vi "Verify Monotonicity.vi"(1 "Data In":string[][](array[string])) -> (0 "Monotonicity":bool)   [LabVIEW 2010]
panel:
  in  "disabled index (col)":i32
  in  "Test Data Array 1":dbl[][](array[numeric])=[[1.0, 20000.0], [2.0, 3000.0], [3.0, 400.0], [4.0, 50.0], [5.0, 6.0], [6.0, 1.0]]
  in  "Test Data Array 2":dbl[][](array[numeric])=[[1.0, 2.0], [2.0, 30.0], [3.0, 400.0], [4.0, 5000.0], [5.0, 60000.0], [6.0, 100000.0]]
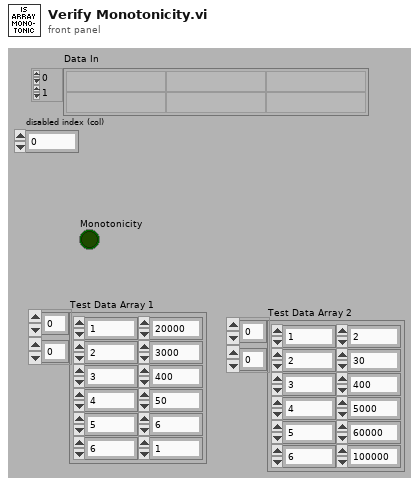
[diagram p1: front panel]
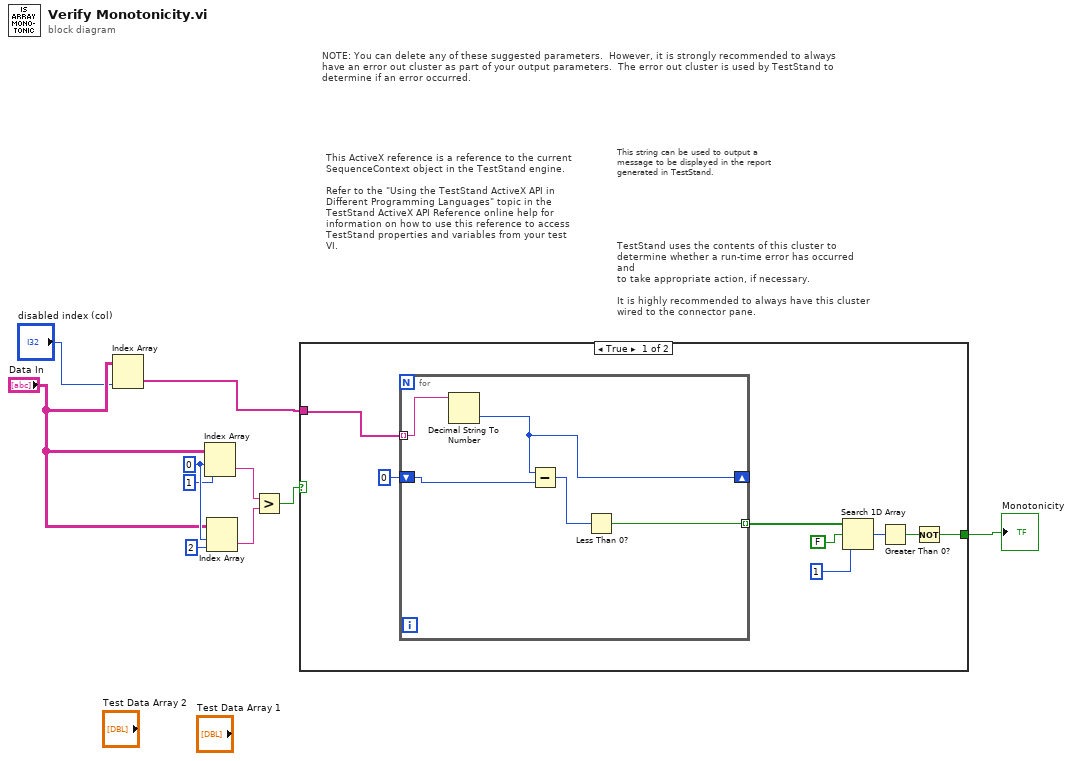
[diagram p0: block diagram]
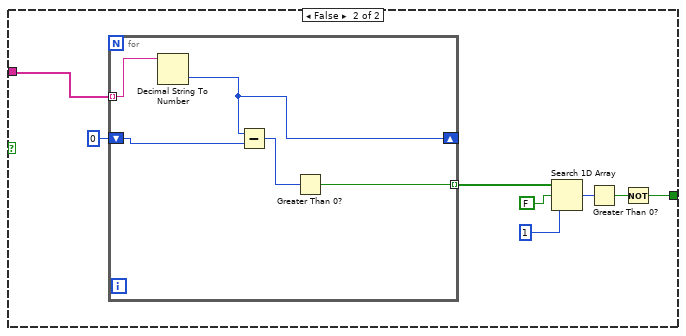
[diagram p2: hidden frame]
diagram:
  w6 = 0 ("index (row)")
  # "TestStand uses the contents of this cluster to\ndetermine whether a run-time error has occurred and\nto take appropriate action, if necessary.\n\nIt is highly recommended to always have this cluster\nwired to the connector pane."
  # "This string can be used to output a\nmessage to be displayed in the report\ngenerated in TestStand."
  # "NOTE: You can delete any of these suggested parameters.  However, it is strongly recommended to always have an error out cluster as part of your output parameters.  The error out cluster is used by TestStand to determine if an error occurred."
  # "This ActiveX reference is a reference to the current\nSequenceContext object in the TestStand engine.\n\nRefer to the \"Using the TestStand ActiveX API in\nDifferent Programming Languages\" topic in the \nTestStand ActiveX API Reference online help for\ninformation on how to use this reference to access\nTestStand properties and variables from your test VI."
  n1 = Index Array(array="Data In", index (col)="disabled index (col)") -> (element=w1:string[])  [unwired: 1 in]
  n2 = Index Array(array="Data In", index (row)=w6, index (col)=1 ("disabled index (col)")) -> (element=w10:string)
  n3 = Index Array(array="Data In", index (row)=w6, index (col)=2 ("disabled index (col)")) -> (element=w9:string)
  n4 = Greater?(x=w10, y=w9) -> (0:w8:bool)
  n5 = case shown="True" w8 {
    tunnel: w1 -> [w18 w31]
    tunnel: [w14 w27] -> w7
    frame True {
      n6 = for {
        tunnel: w18 -> [w21] mode=indexing
        tunnel: [w22] -> w13 mode=indexing
        shift-right: [w20] -> _
        shift-left: 0 -> [w19]
        n7 = Decimal String To Number(string=w21) -> (number=w20:i32)  [unwired: 2 in, 1 out]
        n8 = Subtract(x=w20, y=w19) -> (x-y=w23:i32)
        n9 = Less Than 0?(x=w23) -> (x < 0?=w22:bool)
      }
      n10 = Search 1D Array(1D array=w13, element=FALSE, start index (0)=1) -> (index of element=w16:i32)
      n11 = Greater Than 0?(x=w16) -> (x > 0?=w15:bool)
      n12 = Not(x=w15) -> (.not. x?=w14:bool)
    }
    frame False {
      n13 = for {
        tunnel: w31 -> [w34] mode=indexing
        tunnel: [w35] -> w26 mode=indexing
        shift-right: [w33] -> _
        shift-left: 0 -> [w32]
        n14 = Decimal String To Number(string=w34) -> (number=w33:i32)  [unwired: 2 in, 1 out]
        n15 = Subtract(x=w33, y=w32) -> (x-y=w36:i32)
        n16 = Greater Than 0?(x=w36) -> (x > 0?=w35:bool)
      }
      n17 = Search 1D Array(1D array=w26, element=FALSE, start index (0)=1) -> (index of element=w29:i32)
      n18 = Greater Than 0?(x=w29) -> (x > 0?=w28:bool)
      n19 = Not(x=w28) -> (.not. x?=w27:bool)
    }
  }
  "Monotonicity" <- w7
